vi "Configure Input Sensor Range.vi"(0 "VISA resource name":refnum<visa-resource-name>, 1 "Channel (1)":u16(ring)=1 items=["1"=1, "2"=2, "3"=3, "4"=4, "5"=5, "6"=6, "7"=7, "8"=8, "9"=9, "10"=10, "11"=11, "12"=12, "13"=13, "14"=14, "15"=15, "16"=16, "A (Control Input)"=17], 2 "Excitation Mode (0: Voltage)":u16(ring) items=["Voltage", "Current"], 3 "Excitation Range (5: 200 uV / 100 pA)":u16(ring)=5 items=["2.00 uV / 1.00 pA"=1, "6.32 uV / 3.16 pA"=2, "20.0 uV / 10.0 pA"=3, "63.2 uV / 31.6 pA"=4, "200 uV / 100 pA"=5, "632 uV / 316 pA"=6, "2.00 mV / 1.00 nA"=7, "6.32 mV / 3.16 nA"=8, "20.0 mV / 10.0 nA"=9, "63.2 mV / 31.6 nA"=10, "200 mV / 100 nA"=11, "632 mV / 316 nA"=12, "1.00 uA"=13, "3.16 uA"=14, "10.0 uA"=15, "31.6 uA"=16, "100 uA"=17, "316 uA"=18, "1.00 mA"=19, "3.16 mA"=20, "10.0 mA"=21, "31.6 mA"=22], 4 "Autorange (0: Autorange off)":u16(ring) items=["Autorange off", "Autorange Current", "ROX 102B Autorange"], 5 "error in (no error)":errorcluster, 6 "Resistance Range (17: 200 kOhm)":u16(ring)=17 items=["2.00 mOhm"=1, "6.32 mOhm"=2, "20.0 mOhm"=3, "63.2 mOhm"=4, "200 mOhm"=5, "632 mOhm"=6, "2.00 Ohm"=7, "6.32 Ohm"=8, "20.0 Ohm"=9, "63.2 Ohm"=10, "200 Ohm"=11, "632 Ohm"=12, "2.00 kOhm"=13, "6.32 kOhm"=14, "20.0 kOhm"=15, "63.2 kOhm"=16, "200 kOhm"=17, "632 kOhm"=18, "2.00 MOhm"=19, "6.32 MOhm"=20, "20.0 MOhm"=21, "63.2 MOhm"=22], 7 "Excitation  (T: On)":bool=TRUE, 8 "Preferred Units (2: Ohms)":u16(ring)=2 items=["Kelvin"=1, "Ohms"=2], 9 "Temperature Limit (0 Kelvin)":dbl min=0.0 max=2999.0 step=1.0) -> (14 "VISA resource name out":refnum<visa-resource-name>, 19 "error out":errorcluster)   [LabVIEW 2018, in "Lake Shore 372.lvlib"]
doc: "Configures the Input setup command <B>INTYPE</B> and temperature limit command <B>TLIMIT</B>. Please refer to Model 372 Manual for further explanations.\n\nNotes: \nWhen configuring the control input (A), all parameters must be included, but non-applicable parameters will be ignored. Ie. Resistance Range.\n\nWhen control input A is selected, the control values get modified to represent the appropriate values in for the instruments Excitation Range. Please select the appropriate range for the control input current.\nControl Value Excitation Value \n6 --> 1 \n7 --> 2 \n8 --> 3 \n9 --> 4 \n10 --> 5 \n11 --> 6"
uses:
  Lake Shore 372.lvlib
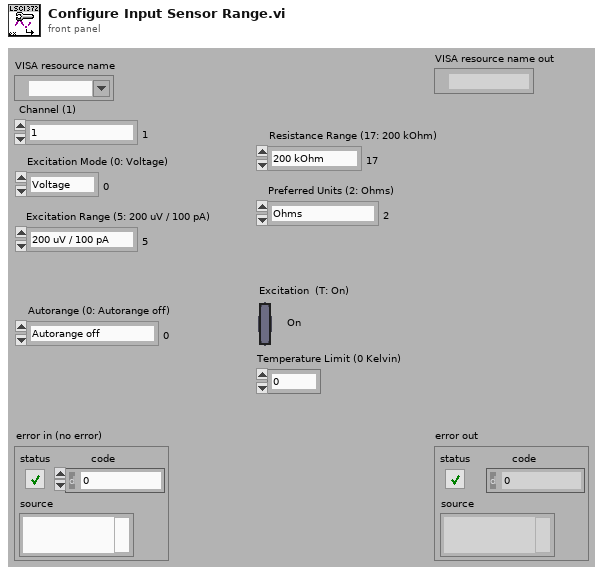
[diagram p1: front panel]
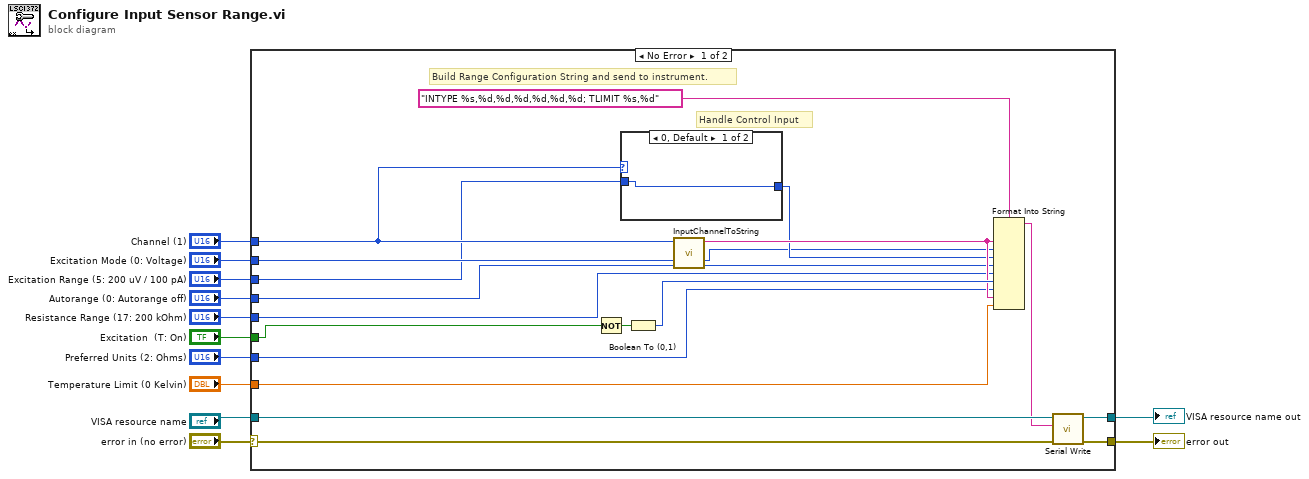
[diagram p0: block diagram]
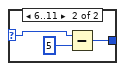
[diagram p3: hidden frame]
diagram:
  n1 = case shown="No Error" "error in (no error)" {
    selector: "error in (no error)" -> [w22 w38]
    tunnel: "VISA resource name" -> [w30 w39]
    tunnel: [w29 w39] -> w11
    tunnel: "Channel (1)" -> [w20 _]
    tunnel: "Temperature Limit (0 Kelvin)" -> [w23 _]
    tunnel: [w21 w38] -> w8
    tunnel: "Excitation Mode (0: Voltage)" -> [w18 _]
    tunnel: "Excitation Range (5: 200 uV / 100 pA)" -> [w17 _]
    tunnel: "Autorange (0: Autorange off)" -> [w16 _]
    tunnel: "Resistance Range (17: 200 kOhm)" -> [w15 _]
    tunnel: "Excitation  (T: On)" -> [w14 _]
    tunnel: "Preferred Units (2: Ohms)" -> [w13 _]
    frame No Error {
      # "Handle Control Input"
      # "Build Range Configuration String and send to instrument."
      n2 = Not(x=w14) -> (.not. x?=w28:bool)
      n3 = case shown="0, Default" w20 {
        tunnel: w17 -> [w31 w33]
        tunnel: [w31 w32] -> w19
        frame 0, Default {
        }
        frame 17 {
          n4 = case shown="0, Default" w33 {
            selector: w33 -> [w34 w37]
            tunnel: [w34 w35] -> w32
            frame 0, Default {
            }
            frame 6..11 {
              n5 = Subtract(x=w37, y=u16 5) -> (x-y=w35:u16)
            }
          }
        }
      }
      n6 = Boolean To (0,1)(Boolean=w28) -> (0, 1=w26:i16)
      n7 = call "InputChannelToString.vi"("Channel (1)"=w20) -> ("Channel Str"=w24:string)  [unwired: 10 in]
      n8 = Format Into String(format string="INTYPE %s,%d,%d,%d,%d,%d,%d; TLIMIT %s,%d", w24, w18, w19, w16, w15, w26, w13, w24, w23) -> (resulting string=w25:string)  [unwired: 2 in, 1 out]
      n9 = call "Serial Write.vi"("error in (no error)"=w22, "Write Buffer (\"\")"=w25, "VISA resource name"=w30) -> ("error out"=w21:errorcluster, "VISA resource name out"=w29:refnum<visa-resource-name>)  [unwired: 6 in, 1 out]
    }
    frame Error {
    }
  }
  "error out" <- w8
  "VISA resource name out" <- w11
